vi "CloseClkRef.vi"(8 "error in (no error)":errorcluster, 11 "NiPxi6683H in":refnum<class "NiPxi6683H.lvclass">) -> (0 "error out":errorcluster, 3 "NiPxi6683H out":refnum<class "NiPxi6683H.lvclass">)   [LabVIEW 2014, in "SyncPlugins.lvlib" / "NiPxi6683H.lvclass"]
uses:
  NiPxi6683H.lvclass
  SyncPluginBase/SyncPluginBase.lvclass/SyncPluginBase.ctl
  NiPxi6682/NiPxi6682.lvclass/NiPxi6682.ctl
  NiPxi6682/Accessors/Read SysHandle.vi
  NiPxi6682/Accessors/Read SysRef.vi
  SyncPluginBase/Accessors/Read Initiated.vi
  <vilib>/nisyscfg/Close (Hardware).vi
  <vilib>/nisyscfg/Close (System).vi
  <vilib>/nisyscfg/nisyscfg.lvlib
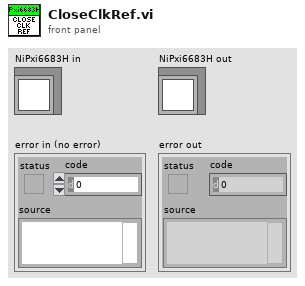
[diagram p1: front panel]
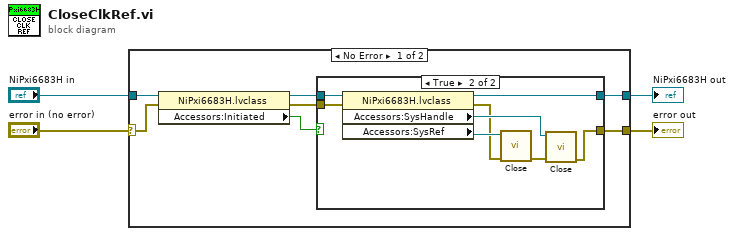
[diagram p0: block diagram]
diagram:
  n1 = case shown="No Error" "error in (no error)" {
    selector: "error in (no error)" -> [w11 w23]
    tunnel: [w6 w23] -> w3
    tunnel: [w5 w22] -> w1
    tunnel: "NiPxi6683H in" -> [w9 w22]
    frame No Error {
      n2 = property class="NiPxi6683H.lvclass"(reference=w9, error in=w11) -> (reference out=w8:refnum<class "NiPxi6683H.lvclass">, error out=w10:errorcluster, "Accessors:Initiated"=w7:bool)
      n3 = case shown="True" w7 {
        tunnel: w10 -> [w12 w17]
        tunnel: w8 -> [w13 w16]
        tunnel: [w12 w15] -> w6
        tunnel: [w13 w14] -> w5
        frame False {
        }
        frame True {
          n4 = property class="NiPxi6683H.lvclass"(reference=w16, error in=w17) -> (reference out=w14:refnum<class "NiPxi6683H.lvclass">, error out=w18:errorcluster, "Accessors:SysHandle"=w20:refnum<k21>, "Accessors:SysRef"=w21:refnum<k20>)
          n5 = call-poly <vilib>:"Close.vi"("error in (no error)"=w18, "Resource in"=w21) -> ("error out"=w19:errorcluster)  [unwired: 9 in]
          n6 = call-poly <vilib>:"Close.vi"("error in (no error)"=w19, "Session in"=w20) -> ("error out"=w15:errorcluster)  [unwired: 9 in]
        }
      }
    }
    frame Error {
    }
  }
  "error out" <- w3
  "NiPxi6683H out" <- w1
